vi "DOE Agilent Tester.vi"() -> ()   [LabVIEW 2020]
uses:
  Drivers/Agilent 34972/Agilent 34970.lvlib
panel:
  in  "VISA Resource Name":refnum<visa-resource-name>
  out "Sorted Data":dbl[](array[numeric])
  out "Instrument IDN":string
  out "Error Message":string
  out "error out":errorcluster
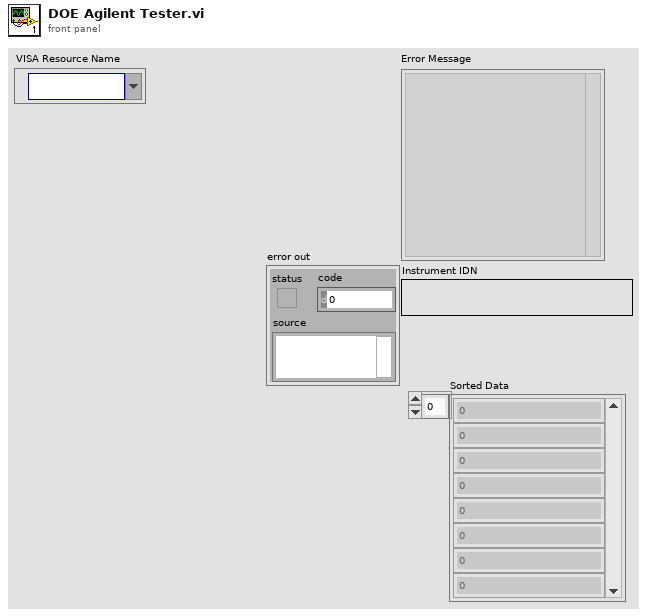
[diagram p1: front panel]
types:
  T1 = enum16{"Temperature", "DC Voltage", "AC Voltage", "DC Current", "AC Current", "Resistance", "4-Wire Resistance", "Frequency", "Period", "Digital", "Totalizer"}
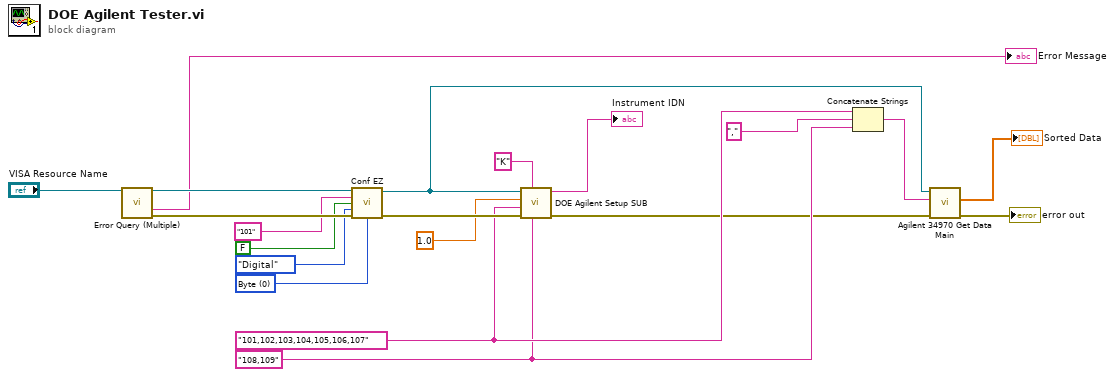
[diagram p0: block diagram]
diagram:
  w7 = "101,102,103,104,105,106,107" ("TC Channels-List")
  w6 = "108,109" ("Analog Channels-List")
  w16 = u16 0 items=["Byte"] ("Digital (0:Byte)")
  n1 = call "Error Query (Multiple).vi"("VISA Resource Name"="VISA Resource Name") -> ("VISA Resource Name Out"=w20:refnum<visa-resource-name>, "Error Message"=→"Error Message":string, "error out"=w19:errorcluster)  [unwired: 11 in, 1 out]
  n2 = call "Conf EZ.vi"("VISA Resource Name"=w20, "Channel List(empty)"="101", "Set/Check (F:Set)"=FALSE, "Measurement (1:DC Volt)"=T1."Digital", "error in (no error)"=w19, "Digital (0:Byte)"=w16) -> ("VISA Resource Name Out"=w2:refnum<visa-resource-name>, "error out"=w13:errorcluster)  [unwired: 7 in, 1 out]
  n3 = call "DOE Agilent Setup SUB.vi"("Analog Channels-List"=w6, "TC Type (K,J,T)"="K", "error in (no error)"=w13, "TC Channels-List"=w7, "Agilent Gain"=1.0, "VISA Refnum in"=w2) -> ("error out"=w4:errorcluster, "Instrument IDN"=→"Instrument IDN":string)  [unwired: 3 in, 1 out]
  n4 = Concatenate Strings(w7, "," ("string"), w6) -> (w9:string)
  n5 = call "Agilent 34970 Get Data Main.vi"("error in (no error)"=w4, "Analog Channels-List"=w9, "VISA Refnum in"=w2) -> ("error out"=→"error out":errorcluster, "Sorted Data"=→"Sorted Data":dbl[])  [unwired: 3 in, 4 out]
